vi "close.vi"(8 "error in":errorcluster) -> (0 "error out":errorcluster)   [LabVIEW 2017]
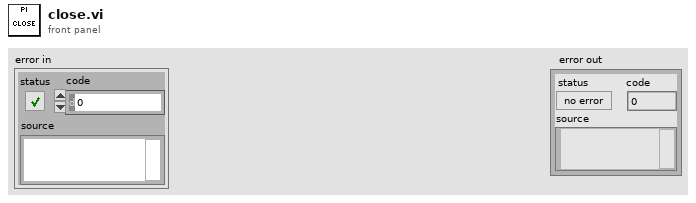
[diagram p1: front panel]
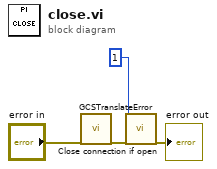
[diagram p0: block diagram]
diagram:
  n1 = call "GCSTranslateError.vi"("error in"="error in") -> ("error out"=w4:errorcluster)  [unwired: 18 out]
  n2 = call "Close connection if open.vi"("System no."=1, "error in"=w4) -> ("error out"=→"error out":errorcluster)  [unwired: 1 in, 16 out]
